vi "Host Image Acquisition Module.vi"(8 "error in":errorcluster, 11 "Operation":T3) -> (0 "error out":errorcluster, 1 "Image Acquired":bool, 2 "Acq In Progress":bool, 3 "Image":T2(plugin-control), 4 "DMA Write Timeout":bool, 6 "Number of Elements to Write Host DMA":u32, 7 "Number of Elements to Read Cam Data":u32)   [LabVIEW 2013]
uses:
  Host Image Acquisition Module Enum.ctl
  Acquisition Settings Cluster.ctl
  <vilib>/vision/Image Controls.llb/IMAQ Image.ctl
  Image Acquisition Settings FG Enum.ctl
  Common/CL Configuration.ctl
  Common/CL Signal Mapping.ctl
  System Status/Status FG Enum.ctl
  Image Processing/Mask ROI FG Enum.ctl
  <vilib>/rvi/interface/common/niFpgaWaitOnOcc.vi
  <vilib>/FPGAPlugInAG/PCIe-1473R/niLvFpga_Reset_PCIe-1473R.vi
  <vilib>/Utility/error.llb/Error Cluster From Error Code.vi
  <vilib>/rvi/errors/niLvFpgaAdjustHostInterfaceError.vi
  <vilib>/FPGAPlugInAG/PCIe-1473R/niLvFpga_Run_PCIe-1473R.vi
  fifodebug.vi
  Globals/Average Sector Data.vi
  <vilib>/FPGAPlugInAG/PCIe-1473R/niLvFpga_Close_PCIe-1473R.vi
  <vilib>/rvi/interface/nirviMethod/nirviMethod.xnode
  FGs/FPGA_Reference.ctl
  FPGA Bitfiles/8-Tap8-bitCamera_FPGATarget_8-Tap8-bit_Serial_Server.lvbitx
  <vilib>/rvi/interface/nirviReadWriteControl/nirviReadWriteControl.xnode
  FPGA/Sector/Accumulate/Sector Parameter Cluster.ctl
  <vilib>/rvi/interface/nirviCloseFPGA/nirviCloseFPGA.xnode
  Common/Timing/Timing Lib.lvlib
  <vilib>/rvi/errors/niLvFpgaMergeErrorWithErrorCode.vi
  NiFpgaLv.dll
  <vilib>/FPGAPlugInAG/PCIe-1473R/niLvFpga_ReadFifo_PCIe-1473R.vi
  <vilib>/FPGAPlugInAG/PCIe-1473R/niLvFpga_ConfigureFifo_PCIe-1473R.vi
  <vilib>/FPGAPlugInAG/PCIe-1473R/niLvFpga_StartFifo_PCIe-1473R.vi
panel:
  out "Actual Depth":u32
  out "Target Sim TO":bool
  out "Cam Data Timeout":bool
  out "Sector FIFO Timeout":bool
  out "Host DMA Timeout":bool
  out "Image Data":u64[](array[numeric])
  out "Elements Remaining":u32
  out "Words per image":u32
  out "Num Frames read":u32
  out "DMA Words per Image":u32
  out "Acquire":bool
  in  "Acquisition Settings Cluster":T1={"Image Width"=2040, "Image Height"=1088, "Frames To Acquire"=0, "Signal Mapping"=enum."Basler 10-tap", "DMA Buffer Size\n(In Images)"=64} {"Image Height" max=65535; "Image Width" max=65535 step=40}
  out "Buffer Size":u32
  out "Acq'd Frame Width":u32=2040
  in  "Start Serial Server":bool
  out "Frames Acq'd":u32=1
  out "Acq'd Frame Height":u32=1088
  out "Initialized":bool
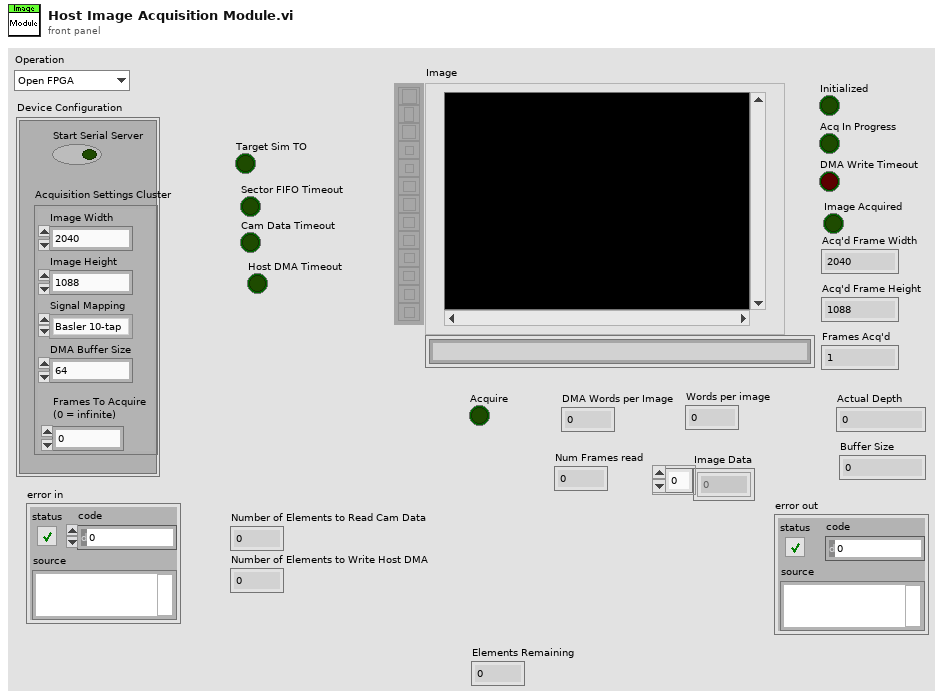
[diagram p1: front panel]
types:
  T1 = typedef "Acquisition Settings Cluster.ctl" = cluster{"Image Width":u32, "Image Height":u32, "Frames To Acquire":u32, "Signal Mapping":enum8{"Standard", "Basler 10-tap", "Vosskühler 10-tap"}, "DMA Buffer Size\n(In Images)":u32}
  T2 = typedef "IMAQ Image.ctl" = refnum<image>
  T3 = typedef "Host Image Acquisition Module Enum.ctl" = enum16{"Open FPGA", "Initialize DMA FIFO", "Load Sim Images", "Initialize Acquisition", "Update Sector Parameters", "Start Acquisition", "Aquire Image", "Read Averages", "Cancel Acquisition", "Close FPGA"}
  T4 = typedef "CL Signal Mapping.ctl" = enum8{"Standard", "Basler 10-tap", "Vosskühler 10-tap"}
  T5 = typedef "CL Configuration.ctl" = enum8{"Base", "Medium", "Full"}
  T6 = typedef "Image Acquisition Settings FG Enum.ctl" = enum16{"Read", "Write"}
  T7 = typedef "Status FG Enum.ctl" = enum16{"Reset", "Read", "Write"}
  T8 = typedef "Mask ROI FG Enum.ctl" = enum16{"Read", "Write"}
  T9 = enum16{"big-endian, network order", "native, host order", "little-endian"}
  T10 = typedef "FPGA_Reference.ctl" = refnum<k20>
  T11 = typedef "Mask ROI Cluster.ctl" = cluster{"left annulus":T12, "right annulus":T12, "Threshold Range":cluster{"Lower value":dbl, "Upper value":dbl}, "[Avg BG]":u8[], "Number of Sectors":u8, "Left ROI":T13, "Right ROI":T13, "Left Start Angle Duty Cycle":fxp<+,8,0>, "Left End Angle Duty Cycle":fxp<+,8,0>, "Right End Angle Duty Cycle":fxp<+,8,0>, "Right Start Angle Duty Cycle":fxp<+,8,0>, "[Sector ROIs]":T13[]}
  T12 = typedef "IMAQ Circle" = cluster{"Center X":i32, "Center Y":i32, "Inner Radius":i32, "Outer Radius":i32, "Start Angle":dbl, "End Angle":dbl}
  T13 = typedef "ROI Descriptor" = cluster{"Global Rectangle":i32[], "Contours":cluster{"ID":enum32{"External", "Internal"}, "Type":u32, "Coordinates":i32[]}[]}
  T14 = typedef "Sector Parameter Cluster.ctl" = cluster{"Start Angle":fxp<+/-,17,2>, "End Angle":fxp<+/-,17,2>, "Inner Radius":u16, "Outter Radius":u16, "Hinge X":u16, "Hinge Y":u16, "NumWingSectors":u8}
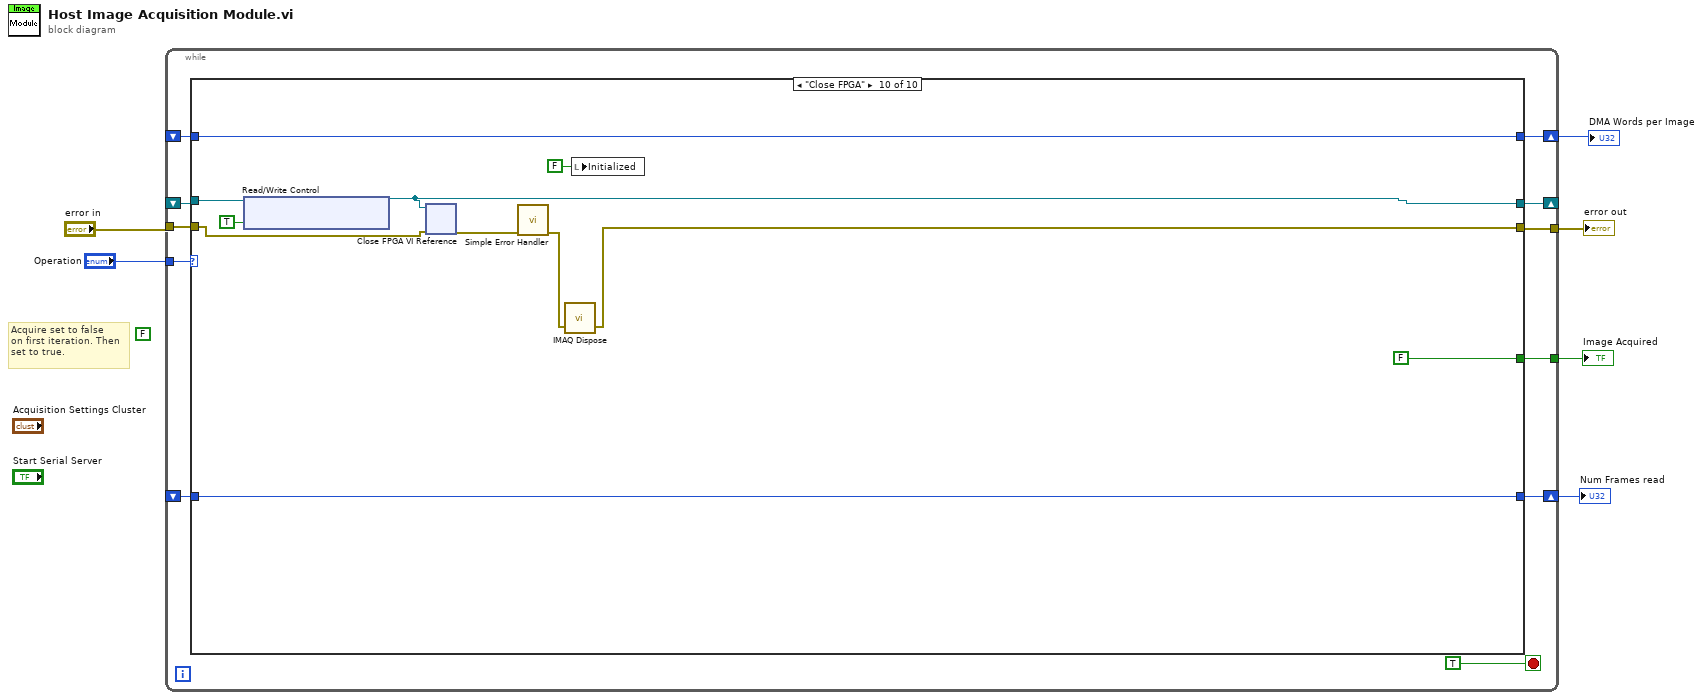
[diagram p0: block diagram]
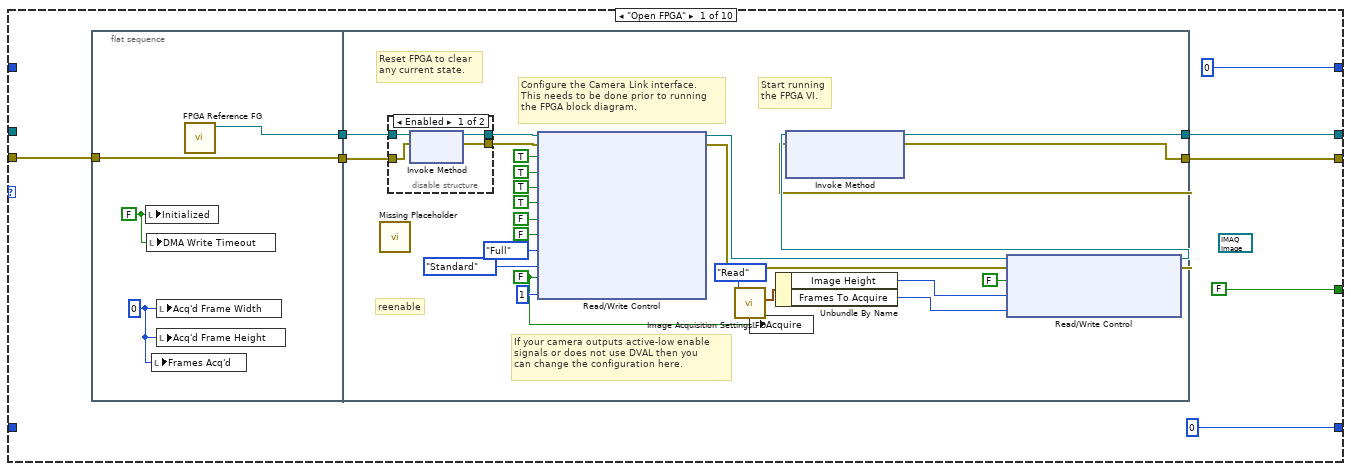
[diagram p2: hidden frame]
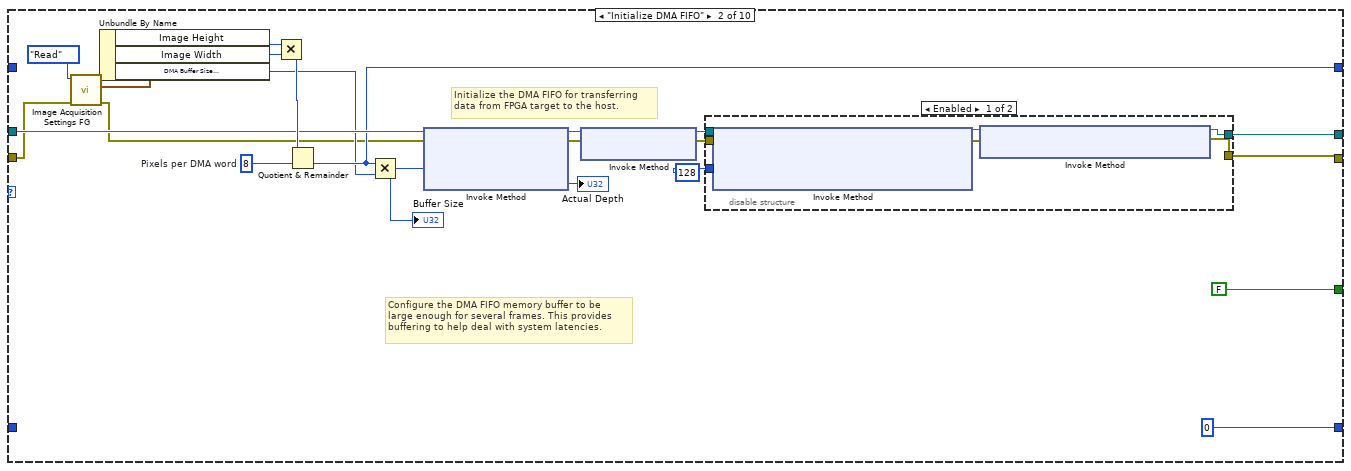
[diagram p4: hidden frame]
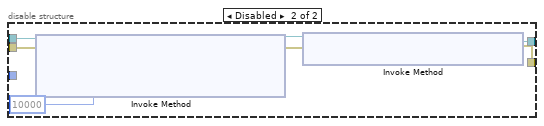
[diagram p5: hidden frame]
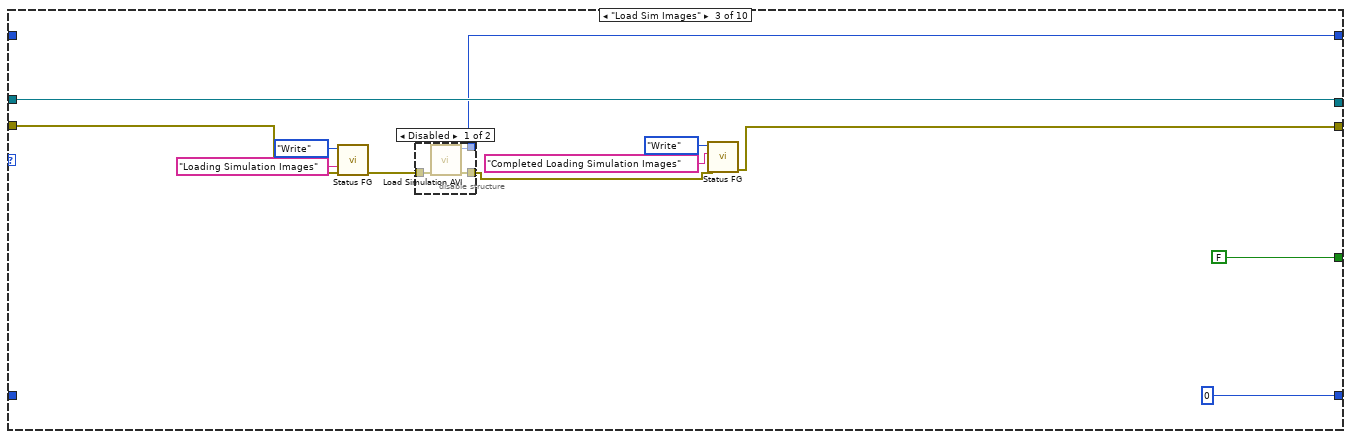
[diagram p6: hidden frame]
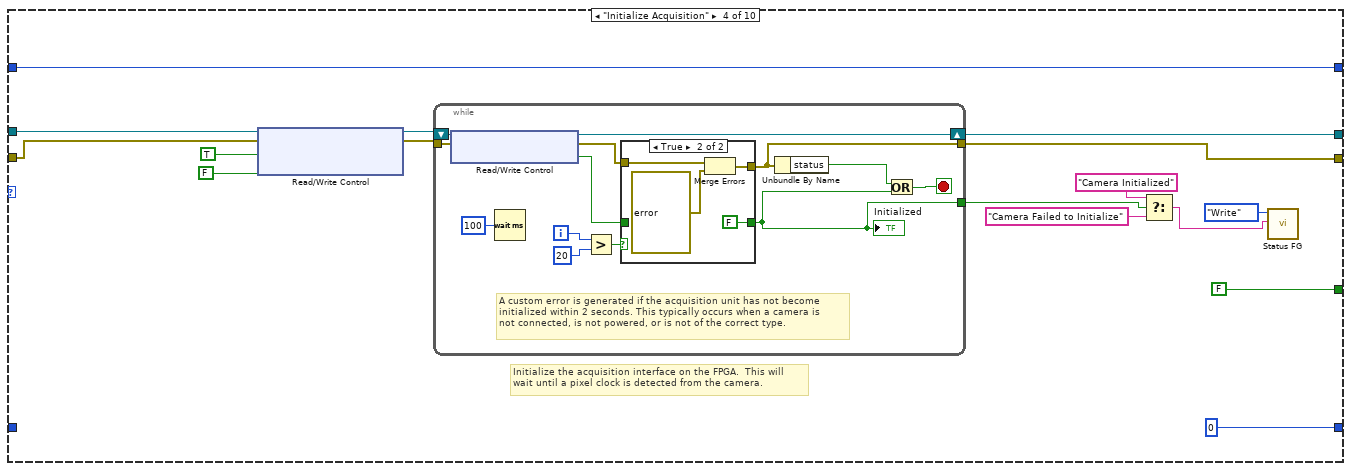
[diagram p8: hidden frame]
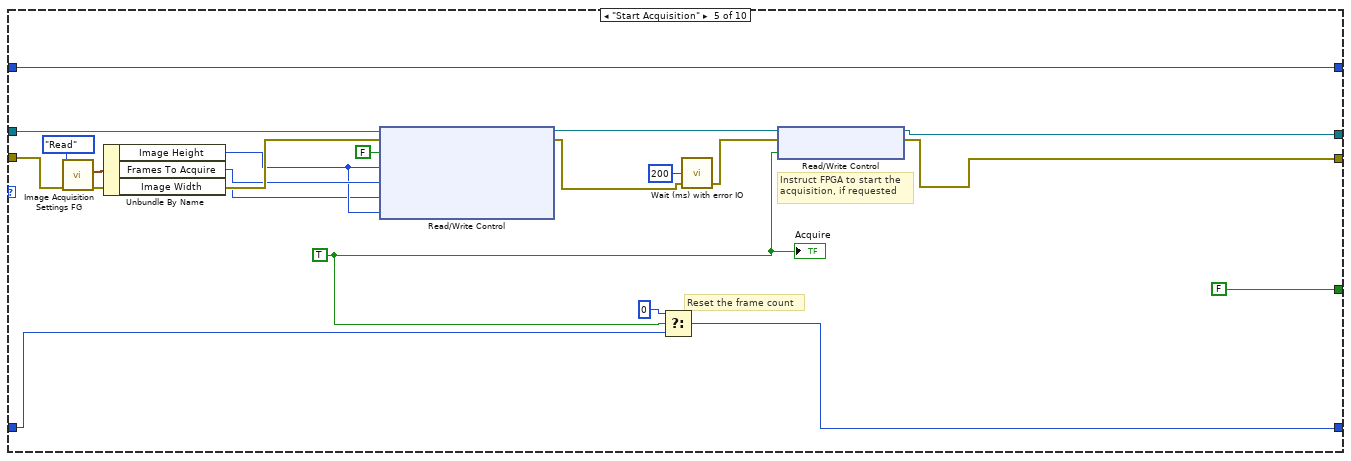
[diagram p10: hidden frame]
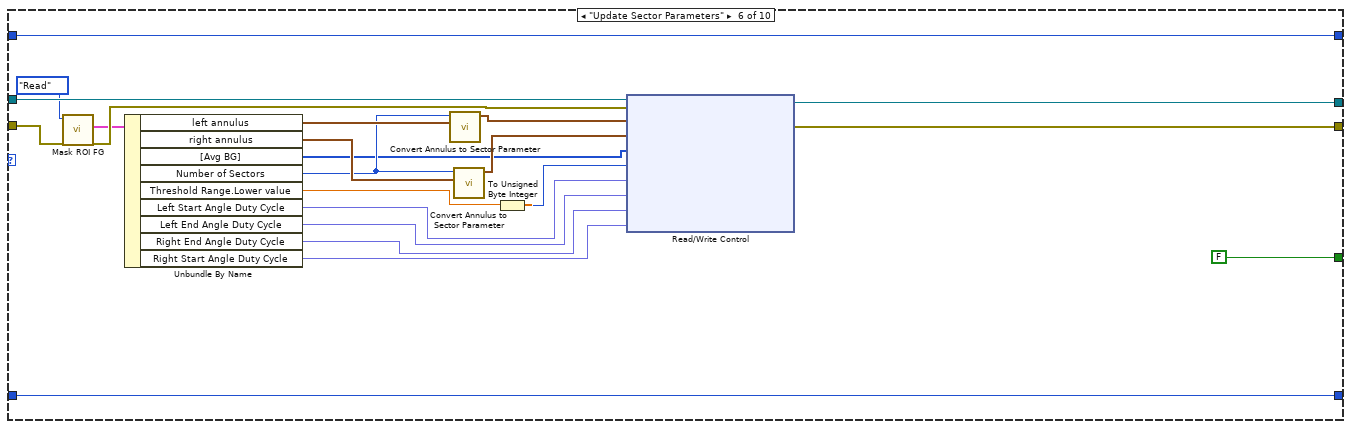
[diagram p11: hidden frame]
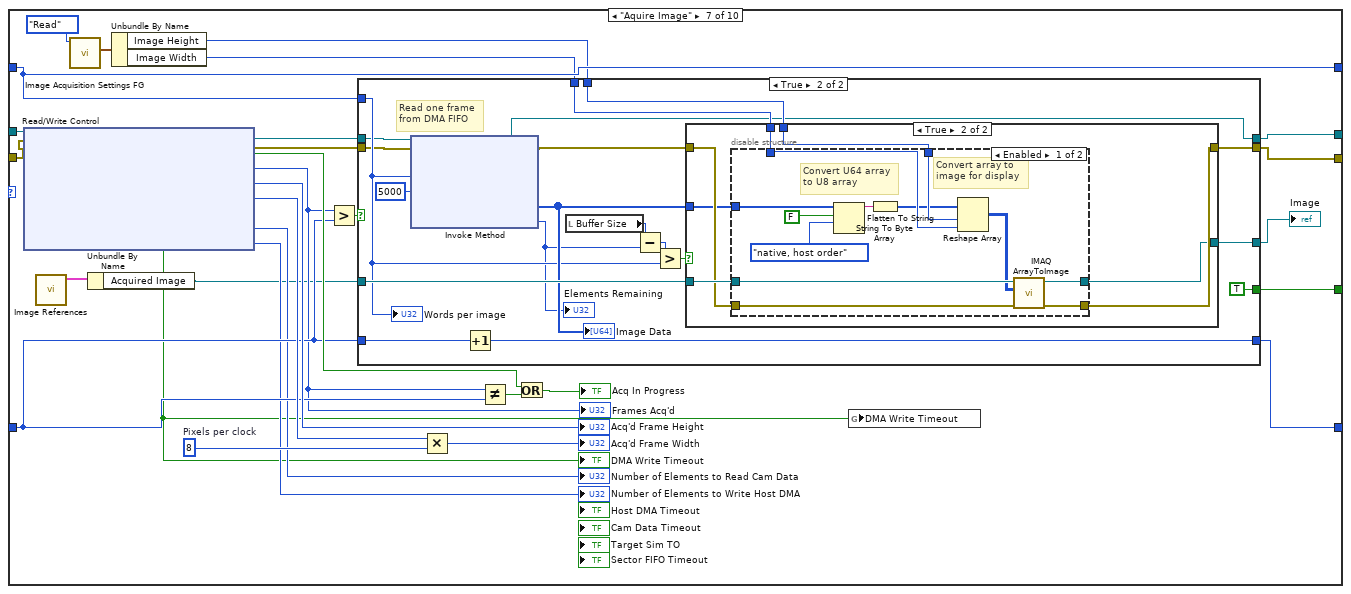
[diagram p12: hidden frame]
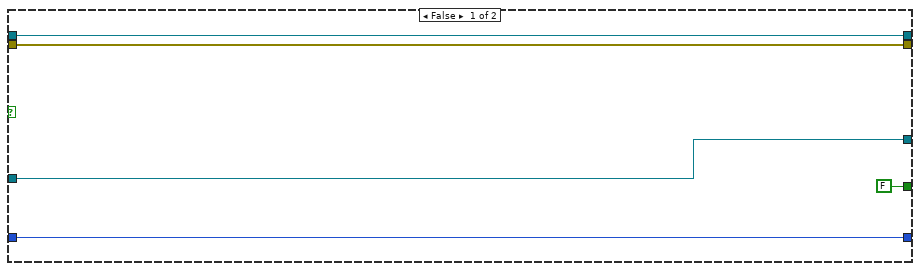
[diagram p13: hidden frame]
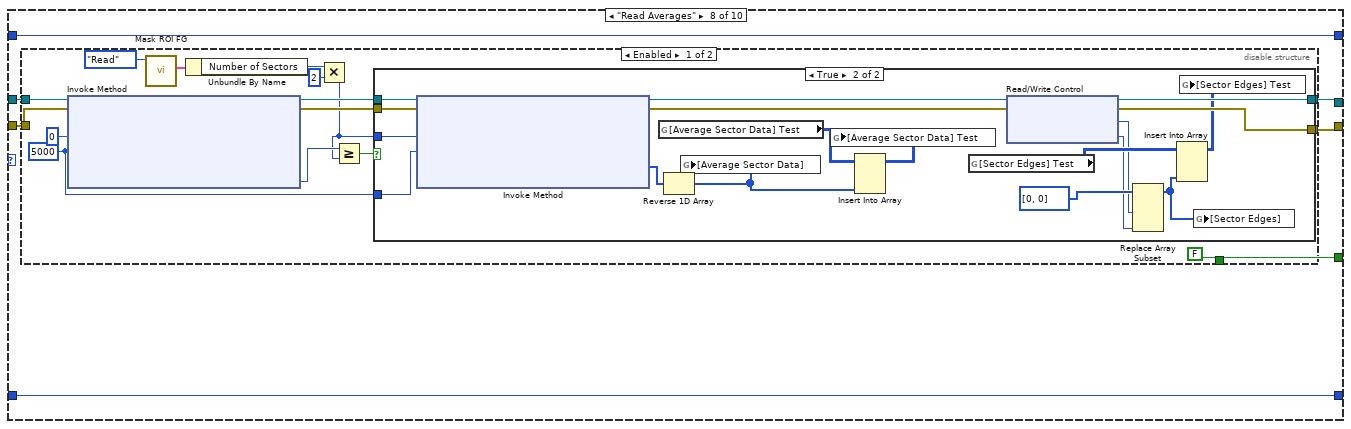
[diagram p16: hidden frame]
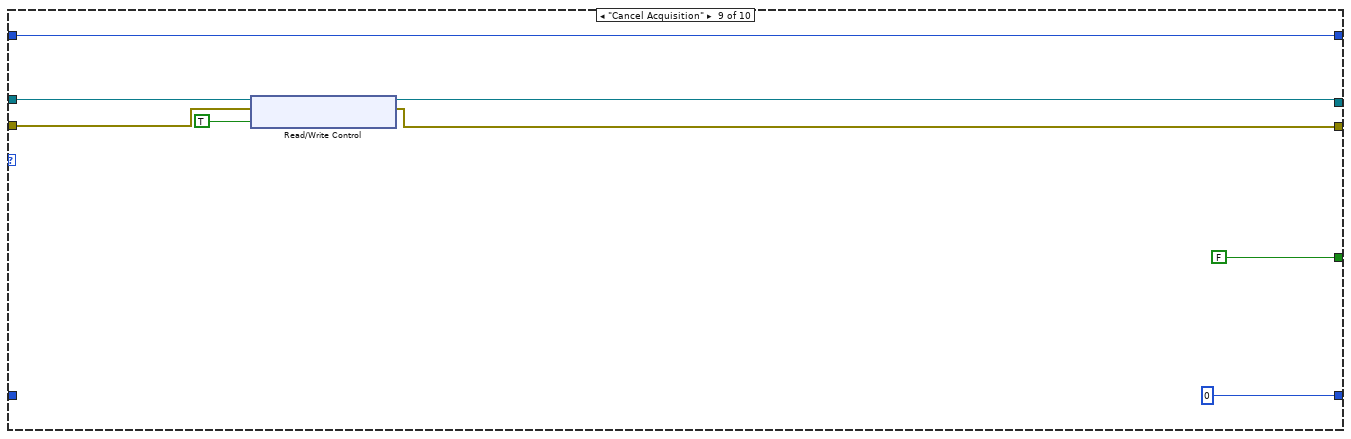
[diagram p19: hidden frame]
diagram:
  (unwired) FALSE ("Acquire")
  # "Acquire set to false\non first iteration. Then\nset to true."
  n1 = while {
    shift-right: [w16] -> _
    shift-left: _ -> [w12]
    tunnel: "error in" -> [w15]
    tunnel: "Operation" -> [w14]
    tunnel: [w13] -> w4
    shift-right: [w11] -> w3
    shift-left: _ -> [w10]
    shift-right: [w9] -> w2
    shift-left: _ -> [w8]
    tunnel: [w7] -> w1
    stop <- TRUE stop-if-true
    n2 = case shown="\"Close FPGA\"" w14 {
      tunnel: w15 -> [w25 w72 w104 w119 w163 w188 w203 w267 w316 w321]
      tunnel: [w24 w66 w107 w124 w157 w184 w218 w272 w317 w322] -> w16
      tunnel: [w23 w61 w98 w120 w156 w185 w217 w268 w315 w327] -> w13
      tunnel: w12 -> [_ w77 w107 w125 w164 w190 w219 w273 w319 w324]
      tunnel: [u32 0 w76 w106 w123 w159 w189 w212 w271 w314 w325] -> w11
      tunnel: w10 -> [_ _ _ w123 w159 w189 w212 w271 w314 w325]
      tunnel: [u32 0 u32 0 u32 0 u32 0 w160 w183 w216 w270 u32 0 w326] -> w9
      tunnel: w8 -> [_ _ _ _ w161 w183 w201 w270 _ w326]
      tunnel: [FALSE ("Image Acquired") FALSE ("Image Acquired") FALSE ("Image Acquired") FALSE ("Image Acquired") FALSE ("Image Acquired") FALSE ("Image Acquired") w197 w269 FALSE ("Image Acquired") FALSE ("Image Acquired")] -> w7
      frame "Open FPGA" {
        (unwired) T2 refnum ("New Image")
        n3 = flat-sequence {
          tunnel: w25 -> [w26]
          tunnel: [w27] -> w22
          tunnel: [w26] -> w21
          tunnel: [w43] -> w23
          tunnel: [w44] -> w24
          tunnel: w22 -> [w47]
          tunnel: w21 -> [w45]
          frame #0 {
            w28 = u32 0 ("Acq'd Frame Width")
            w29 = FALSE ("Initialized")
            n4 = local write "Initialized"(w29) -> ()
            n5 = local write "DMA Write Timeout"(w29) -> ()
            n6 = local write "Frames Acq'd"(w28) -> ()
            n7 = local write "Acq'd Frame Width"(w28) -> ()
            n8 = local write "Acq'd Frame Height"(w28) -> ()
            n9 = call "FPGA Reference FG.vi"() -> ("FPGA VI Reference Out"=w27:T10)  [unwired: 11 in]
          }
          frame #1 {
            w41 = FALSE ("Acq Control.Acquire")
            # "reenable"
            # "If your camera outputs active-low enable\nsignals or does not use DVAL then you \ncan change the configuration here."
            # "Start running\nthe FPGA VI."
            # "Reset FPGA to clear\nany current state."
            # "Configure the Camera Link interface.\nThis needs to be done prior to running\nthe FPGA block diagram."
            n10 = call "Missing Placeholder.vi"() -> ()  [unwired: 12 in]
            n11 = disable-structure shown="Enabled" {
              disable-tunnel: [w58 w60] -> w49
              disable-tunnel: [w57 w59] -> w48
              disable-tunnel: w47 -> [w56 w60]
              disable-tunnel: w45 -> [w55 w59]
              frame Enabled {
                n12 = xnode "Invoke Method"("FPGA VI Reference In"=w56, "error in"=w55) -> ("FPGA VI Reference Out"=w58:T10, "error out"=w57:errorcluster)
              }
              frame Disabled {
              }
            }
            n13 = xnode "Read/Write Control"("FPGA VI Reference In"=w49, "error in"=w48, "CL Config.FVAL Active High"=TRUE ("IO Module Config.CL FVAL Active High"), "CL Config.LVAL Active High"=TRUE ("IO Module Config.CL LVAL Active High"), "CL Config.DVAL Active High"=TRUE ("IO Module Config.CL DVAL Active High"), "CL Config.Spare Active High"=TRUE ("IO Module Config.CL Spare Active High"), "CL Config.Line Scan"=FALSE, "Acq Control.Ignore DVAL"=FALSE ("CL Config.Line Scan"), "CL Config.Configuration"=CL_Configuration."Full", "CL Config.Signal Mapping"=CL_Signal_Mapping."Standard", "Acq Control.Acquire"=w41, "# of Frames to Average"=u8 1) -> ("FPGA VI Reference Out"=w36:T10, "error out"=w34:errorcluster)
            n14 = call "Image Acquisition Settings FG.vi"("Operation"=Image_Acquisition_Settings_FG_Enum."Read") -> ("Acquisition Settings Out"=w40:T1)  [unwired: 9 in, 1 out]
            n15 = local write "Acquire"(w41) -> ()
            n16 = Unbundle By Name(w40) -> ("Image Height"=w38:u32, "Frames To Acquire"=w32:u32)
            n17 = xnode "Read/Write Control"("FPGA VI Reference In"=w36, "error in"=w34, "Acq Control.Cancel Acq"=FALSE, "Acq Control.Line Scan Height"=w38, "Acq Control.Frames To Acq"=w32) -> ("FPGA VI Reference Out"=w35:T10, "error out"=w33:errorcluster)
            n18 = xnode "Invoke Method"("FPGA VI Reference In"=w35, "error in"=w33) -> ("FPGA VI Reference Out"=w44:T10, "error out"=w43:errorcluster)  [unwired: 1 in]
          }
        }
      }
      frame "Initialize DMA FIFO" {
        w79 = u32 8  # Pixels per DMA word
        # "Configure the DMA FIFO memory buffer to be\nlarge enough for several frames. This provides\nbuffering to help deal with system latencies."
        # "Initialize the DMA FIFO for transferring\ndata from FPGA target to the host."
        n19 = call "Image Acquisition Settings FG.vi"("error in (no error)"=w72, "Operation"=Image_Acquisition_Settings_FG_Enum."Read") -> ("error out"=w67:errorcluster, "Acquisition Settings Out"=w73:T1)  [unwired: 8 in]
        n20 = Unbundle By Name(w73) -> ("Image Height"=w71:u32, "Image Width"=w70:u32, "DMA Buffer Size\n(In Images)"=w69:u32)
        n21 = Multiply(x=w71, y=w70) -> (x*y=w78:u32)
        n22 = Quotient & Remainder(x=w78, y=w79) -> (floor(x/y)=w76:u32)  [unwired: 1 out]
        n23 = Multiply(x=w76, y=w69) -> (x*y=w80:u32)
        "Buffer Size" <- w80
        n24 = xnode "Invoke Method"("FPGA VI Reference In"=w77, "error in"=w67, "Requested Depth"=w80) -> ("FPGA VI Reference Out"=w82:T10, "error out"=w81:errorcluster, "Actual Depth"=→"Actual Depth":u32)
        n25 = xnode "Invoke Method"("FPGA VI Reference In"=w82, "error in"=w81) -> ("FPGA VI Reference Out"=w64:T10, "error out"=w62:errorcluster)
        n26 = disable-structure shown="Enabled" {
          disable-tunnel: u32 128 ("Requested Depth") -> [w89 _]
          disable-tunnel: [w88 w96] -> w66
          disable-tunnel: w64 -> [w87 w95]
          disable-tunnel: w62 -> [w86 w94]
          disable-tunnel: [w83 w91] -> w61
          frame Enabled {
            n27 = xnode "Invoke Method"("FPGA VI Reference In"=w87, "error in"=w86, "Requested Depth"=w89) -> ("FPGA VI Reference Out"=w85:T10, "error out"=w84:errorcluster)  [unwired: 1 out]
            n28 = xnode "Invoke Method"("FPGA VI Reference In"=w85, "error in"=w84) -> ("FPGA VI Reference Out"=w88:T10, "error out"=w83:errorcluster)
          }
          frame Disabled {
            n29 = xnode "Invoke Method"("FPGA VI Reference In"=w95, "error in"=w94, "Requested Depth"=u32 10000) -> ("FPGA VI Reference Out"=w93:T10, "error out"=w92:errorcluster)  [unwired: 1 out]
            n30 = xnode "Invoke Method"("FPGA VI Reference In"=w93, "error in"=w92) -> ("FPGA VI Reference Out"=w96:T10, "error out"=w91:errorcluster)
          }
        }
      }
      frame "Load Sim Images" {
        n31 = call "Status FG.vi"("error in (no error)"=w104, "Status In"="Loading Simulation Images", "Operation"=Status_FG_Enum."Write") -> ("error out"=w103:errorcluster)  [unwired: 7 in, 1 out]
        n32 = disable-structure shown="Disabled" {
          disable-tunnel: [w111 _] -> w106
          disable-tunnel: w103 -> [w110 w112]
          disable-tunnel: [w109 w112] -> w99
          frame Disabled {
            n33 = call "Load Simulation AVI.vi"("error in (no error)"=w110) -> ("error out"=w109:errorcluster, "Words per image"=w111:u32)  [unwired: 9 in]
          }
          frame Enabled {
          }
        }
        n34 = call "Status FG.vi"("error in (no error)"=w99, "Status In"="Completed Loading Simulation Images", "Operation"=Status_FG_Enum."Write") -> ("error out"=w98:errorcluster)  [unwired: 7 in, 1 out]
      }
      frame "Initialize Acquisition" {
        # "Initialize the acquisition interface on the FPGA.  This will\nwait until a pixel clock is detected from the camera."
        n35 = xnode "Read/Write Control"("FPGA VI Reference In"=w125, "error in"=w119, "Acq Control.Initialize"=TRUE ("Arm Acquisition"), "Acq Control.Cancel Acq"=FALSE) -> ("FPGA VI Reference Out"=w128:T10, "error out"=w127:errorcluster)
        n36 = while {
          tunnel: w127 -> [w136]
          tunnel: [w138] -> w120
          shift-right: [w135] -> w124
          shift-left: w128 -> [w137]
          tunnel: [w129] -> w115
          i -> [w131]
          stop <- w141 stop-if-true
          # "A custom error is generated if the acquisition unit has not become\ninitialized within 2 seconds. This typically occurs when a camera is\nnot connected, is not powered, or is not of the correct type."
          n37 = xnode "Read/Write Control"("FPGA VI Reference In"=w137, "error in"=w136) -> ("FPGA VI Reference Out"=w135:T10, "error out"=w134:errorcluster, "Acq Status.Initialized"=w133:bool)
          n38 = Wait (ms)(milliseconds to wait=u32 100) -> ()  [unwired: 1 out]
          n39 = Greater?(x=w131, y=20) -> (0:w132:bool)
          n40 = case shown="True" w132 {
            tunnel: [w143 FALSE] -> w129
            tunnel: w133 -> [w143 _]
            tunnel: w134 -> [w142 w145]
            tunnel: [w142 w147] -> w138
            frame False {
            }
            frame True {
              n41 = Merge Errors(w145, errorcluster {"status"=TRUE, "code"=-8999, "source"="Acquisition Initialization: This error typically occurs when a camera is not properly connected, is not powered, or is not of the correct type."} ("error in")) -> (w147:errorcluster)
            }
          }
          "Initialized" <- w129
          n42 = Unbundle By Name(w138) -> ("status"=w140:bool)
          n43 = Or(x=w140, y=w129) -> (x .or. y?=w141:bool)
        }
        n44 = Select(t="Camera Initialized", s=w115, f="Camera Failed to Initialize") -> (s? t:f=w117:string)
        n45 = call "Status FG.vi"("Status In"=w117, "Operation"=Status_FG_Enum."Write") -> ()  [unwired: 8 in, 2 out]
      }
      frame "Start Acquisition" {
        w165 = TRUE ("Acquire")
        # "Reset the frame count"
        # "Instruct FPGA to start the\nacquisition, if requested"
        n46 = call "Image Acquisition Settings FG.vi"("error in (no error)"=w163, "Operation"=Image_Acquisition_Settings_FG_Enum."Read") -> ("error out"=w162:errorcluster, "Acquisition Settings Out"=w168:T1)  [unwired: 8 in]
        n47 = Unbundle By Name(w168) -> ("Image Height"=w149:u32, "Frames To Acquire"=w154:u32, "Image Width"=w148:u32)
        n48 = xnode "Read/Write Control"("FPGA VI Reference In"=w164, "error in"=w162, "Acq Control.Cancel Acq"=FALSE, "Acq Control.Line Scan Height"=w149, "Acq Control.Frames To Acq"=w154, "X Resolution"=w148, "Y Resolution"=w149) -> ("FPGA VI Reference Out"=w153:T10, "error out"=w152:errorcluster)
        n49 = Select(t=u32 0, s=w165, f=w161) -> (s? t:f=w160:u32)
        n50 = call "Wait (ms) with error IO.vi"("error in (no error)"=w152, "milliseconds to wait"=u32 200) -> ("error out"=w151:errorcluster)  [unwired: 3 in]
        n51 = xnode "Read/Write Control"("FPGA VI Reference In"=w153, "error in"=w151, "Acq Control.Acquire"=w165) -> ("FPGA VI Reference Out"=w157:T10, "error out"=w156:errorcluster)
        "Acquire" <- w165
      }
      frame "Update Sector Parameters" {
        n52 = call "Mask ROI FG.vi"("error in (no error)"=w188, "Operation"=Mask_ROI_FG_Enum."Read") -> ("error out"=w187:errorcluster, "Mask ROI Out"=w182:T11)  [unwired: 8 in]
        n53 = Unbundle By Name(w182) -> ("left annulus"=w181:T12, "right annulus"=w179:T12, "[Avg BG]"=w176:u8[], "Number of Sectors"=w178:u8, "Threshold Range.Lower value"=w174:dbl, "Left Start Angle Duty Cycle"=w172:fxp<+,8,0>, "Left End Angle Duty Cycle"=w171:fxp<+,8,0>, "Right End Angle Duty Cycle"=w170:fxp<+,8,0>, "Right Start Angle Duty Cycle"=w169:fxp<+,8,0>)
        n54 = call "Convert Annulus to Sector Parameter.vi"("Annulus"=w181, "NumWingSectors"=w178) -> ("Sector Parameter"=w180:T14)  [unwired: 9 in]
        n55 = call "Convert Annulus to Sector Parameter.vi"("Annulus"=w179, "NumWingSectors"=w178) -> ("Sector Parameter"=w177:T14)  [unwired: 9 in]
        n56 = To Unsigned Byte Integer(number=w174) -> (unsigned 8bit integer=w173:u8)
        n57 = xnode "Read/Write Control"("FPGA VI Reference In"=w190, "error in"=w187, "Sector Parameters Left"=w180, "Sector Parameters Right"=w177, "[Average BG Intensity]"=w176, "Sector Threshold"=w173, "Left Start Angle Duty Cycle"=w172, "Left End Angle Duty Cycle"=w171, "Right End Angle Duty Cycle"=w170, "Right Start Angle Duty Cycle"=w169) -> ("FPGA VI Reference Out"=w184:T10, "error out"=w185:errorcluster)
      }
      frame "Aquire Image" {
        w210 = u32 8  # Pixels per clock
        n58 = xnode "Read/Write Control"("FPGA VI Reference In"=w219, "error in"=w203) -> ("FPGA VI Reference Out"=w215:T10, "error out"=w214:errorcluster, "Acq Status.Acq In Progress"=w202:bool, "Acq Status.Frames Acq'd"=w200:u32, "Acq Status.Lines Per Frame"=→"Acq'd Frame Height":u32, "Acq Status.Clocks Per Line"=w209:u32, "Acq Status.DMA Write Timeout"=w194:bool, "Number of Elements to Read Cam Data"=→"Number of Elements to Read Cam Data":u32, "Number of Elements to Write Host DMA"=→"Number of Elements to Write Host DMA":u32)
        "Frames Acq'd" <- w200
        "DMA Write Timeout" <- w194
        n59 = call "Image References.vi"() -> ("Images"=w193:cluster{"Acquired Image":T2, "Display Image":T2})  [unwired: 10 in, 1 out]
        n60 = call "Image Acquisition Settings FG.vi"("Operation"=Image_Acquisition_Settings_FG_Enum."Read") -> ("Acquisition Settings Out"=w206:T1)  [unwired: 9 in, 1 out]
        n61 = Unbundle By Name(w193) -> ("Acquired Image"=w192:T2)
        n62 = Unbundle By Name(w206) -> ("Image Height"=w205:u32, "Image Width"=w204:u32)
        n63 = Greater?(x=w200, y=w201) -> (0:w213:bool)
        n64 = case shown="True" w213 {
          tunnel: w215 -> [w223 w226]
          tunnel: w214 -> [w222 w227]
          tunnel: w205 -> [_ w243]
          tunnel: w204 -> [_ w242]
          tunnel: w192 -> [w224 w241]
          tunnel: [w222 w239] -> w217
          tunnel: [w223 w238] -> w218
          tunnel: w201 -> [w221 w237]
          tunnel: [w221 w236] -> w216
          tunnel: w212 -> [_ w233]
          tunnel: [w224 w232] -> w191
          tunnel: [FALSE ("Image Acquired") TRUE ("Image Acquired")] -> w197
          frame False {
          }
          frame True {
            # "Read one frame\nfrom DMA FIFO"
            n65 = xnode "Invoke Method"("FPGA VI Reference In"=w226, "error in"=w227, "Number of Elements"=w233, "Timeout (ms)"=5000) -> ("FPGA VI Reference Out"=w238:T10, "error out"=w240:errorcluster, "Data"=w235:u64[], "Elements Remaining"=w230:u32)
            "Elements Remaining" <- w230
            "Image Data" <- w235
            n66 = Increment(x=w237) -> (x+1=w236:u32)
            n67 = local read "Buffer Size"() -> (w231:u32)
            n68 = Subtract(x=w231, y=w230) -> (x-y=w229:u32)
            n69 = Greater?(x=w229, y=w233) -> (0:w234:bool)
            n70 = case shown="True" w234 {
              tunnel: w243 -> [_ w252]
              tunnel: w242 -> [_ w251]
              tunnel: w241 -> [w244 w250]
              tunnel: w240 -> [w245 w249]
              tunnel: [w245 w248] -> w239
              tunnel: w235 -> [_ w247]
              tunnel: [w244 w246] -> w232
              frame False {
                # "Do not display the image if we're\nfalling behind in the acquisition."
              }
              frame True {
                n71 = disable-structure shown="Enabled" {
                  disable-tunnel: w252 -> [w264 _]
                  disable-tunnel: w251 -> [w263 _]
                  disable-tunnel: w250 -> [w262 w266]
                  disable-tunnel: w249 -> [w261 w265]
                  disable-tunnel: [w260 w265] -> w248
                  disable-tunnel: w247 -> [w257 _]
                  disable-tunnel: [w253 w266] -> w246
                  frame Enabled {
                    # "Convert U64 array\nto U8 array"
                    # "Convert array to\nimage for display"
                    n72 = Flatten To String(anything=w257, prepend array or string size? (T)=FALSE, byte order (0:big-endian, network order)=T9."native, host order") -> (data string=w255:string)  [unwired: 1 in, 2 out]
                    n73 = String To Byte Array(string=w255) -> (unsigned byte array=w254:u8[])
                    n74 = Reshape Array(w254, w264, w263) -> (w259:u8[][])
                    n75 = call "IMAQ ArrayToImage"("error in (no error)"=w261, "Image Pixels (U8)"=w259, "Image"=w262) -> ("error out"=w260:errorcluster, "Image Out"=w253:T2)  [unwired: 7 in]
                  }
                  frame Disabled {
                  }
                }
              }
            }
            "Words per image" <- w233
          }
        }
        "Image" <- w191
        n76 = Multiply(x=w209, y=w210) -> (x*y=→"Acq'd Frame Width":u32)
        n77 = Not Equal?(x=w200, y=w201) -> (x != y?=w199:bool)
        n78 = Or(x=w202, y=w199) -> (x .or. y?=→"Acq In Progress":bool)
        n79 = global write "fifodebug.vi" "DMA Write Timeout"(w194) -> ()
      }
      frame "Read Averages" {
        n80 = disable-structure shown="Enabled" {
          disable-tunnel: w273 -> [w289 w311]
          disable-tunnel: [w288 w311] -> w272
          disable-tunnel: [FALSE ("Image Acquired") _] -> w269
          disable-tunnel: [w286 w310] -> w268
          disable-tunnel: w267 -> [w285 w310]
          frame Enabled {
            w281 = 5000 ("Timeout (ms)")
            n81 = xnode "Invoke Method"("FPGA VI Reference In"=w289, "error in"=w285, "Number of Elements"=u32 0, "Timeout (ms)"=w281) -> ("FPGA VI Reference Out"=w283:T10, "error out"=w282:errorcluster, "Elements Remaining"=w276:u32)  [unwired: 1 out]
            n82 = call "Mask ROI FG.vi"("Operation"=Mask_ROI_FG_Enum."Read") -> ("Mask ROI Out"=w279:T11)  [unwired: 9 in, 1 out]
            n83 = Unbundle By Name(w279) -> ("Number of Sectors"=w277:u8)
            n84 = Multiply(x=w277, y=u8 2) -> (x*y=w275:u8)
            n85 = Greater Or Equal?(x=w276, y=w275) -> (x >= y?=w278:bool)
            n86 = case shown="True" w278 {
              tunnel: w283 -> [w291 w309]
              tunnel: w282 -> [w290 w308]
              tunnel: w281 -> [_ w307]
              tunnel: [w291 w300] -> w288
              tunnel: [w290 w301] -> w286
              tunnel: w275 -> [_ w306]
              frame False {
              }
              frame True {
                n87 = xnode "Invoke Method"("FPGA VI Reference In"=w309, "error in"=w308, "Number of Elements"=w306, "Timeout (ms)"=w307) -> ("FPGA VI Reference Out"=w303:T10, "error out"=w302:errorcluster, "Data"=w297:u8[])  [unwired: 1 out]
                n88 = global read "Average Sector Data.vi" "[Average Sector Data] Test"() -> (w305:u8[][])
                n89 = Reverse 1D Array(array=w297) -> (reversed array=w296:u8[])
                n90 = global write "Average Sector Data.vi" "[Average Sector Data]"(w296) -> ()
                n91 = Insert Into Array(array=w305, new element=w296) -> (w304:u8[][])  [unwired: 2 in]
                n92 = global write "Average Sector Data.vi" "[Average Sector Data] Test"(w304) -> ()
                n93 = global read "Average Sector Data.vi" "[Sector Edges] Test"() -> (w299:u8[][])
                n94 = xnode "Read/Write Control"("FPGA VI Reference In"=w303, "error in"=w302) -> ("FPGA VI Reference Out"=w300:T10, "error out"=w301:errorcluster, "Right Sector Edge"=w294:u8, "Left Sector Edge"=w293:u8)
                n95 = Replace Array Subset(array=u8[] [0, 0] ("[Sector Edges]"), new element #1=w294, new element #2=w293) -> (w292:u8[])  [unwired: 2 in]
                n96 = Insert Into Array(array=w299, new element=w292) -> (w298:u8[][])  [unwired: 2 in]
                n97 = global write "Average Sector Data.vi" "[Sector Edges] Test"(w298) -> ()
                n98 = global write "Average Sector Data.vi" "[Sector Edges]"(w292) -> ()
              }
            }
          }
          frame Disabled {
          }
        }
      }
      frame "Cancel Acquisition" {
        n99 = xnode "Read/Write Control"("FPGA VI Reference In"=w319, "error in"=w316, "Acq Control.Cancel Acq"=TRUE) -> ("FPGA VI Reference Out"=w317:T10, "error out"=w315:errorcluster)
      }
      frame "Close FPGA" {
        n100 = xnode "Read/Write Control"("FPGA VI Reference In"=w324, "Acq Control.Cancel Acq"=TRUE) -> ("FPGA VI Reference Out"=w322:T10)  [unwired: 1 in, 1 out]
        n101 = xnode "Close FPGA VI Reference"("FPGA VI Reference In"=w322, "error in"=w321) -> ("error out"=w330:errorcluster)
        n102 = call <vilib>:"Simple Error Handler.vi"("error in (no error)"=w330) -> ("error out"=w328:errorcluster)  [unwired: 4 in, 4 out]
        n103 = call "IMAQ Dispose"("error in (no error)"=w328) -> ("error out"=w327:errorcluster)  [unwired: 5 in]
        n104 = local write "Initialized"(FALSE ("Initialized")) -> ()
      }
    }
  }
  "error out" <- w4
  "DMA Words per Image" <- w3
  "Num Frames read" <- w2
  "Image Acquired" <- w1
